vi "ADO Fields Get Count.vi"(8 "error in (no error)":errorcluster, 11 "Fields In":refnum<k7>) -> (0 "error out":errorcluster, 2 "Count":i32, 3 "Fields Out":refnum<k7>)   [LabVIEW 2013]
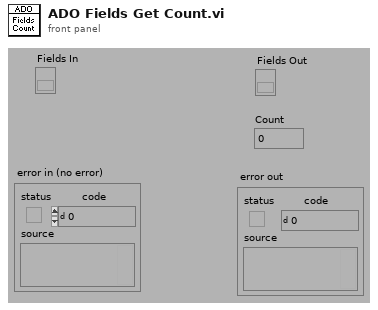
[diagram p1: front panel]
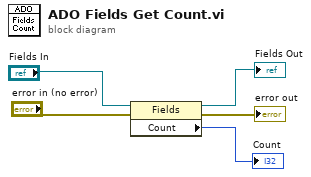
[diagram p0: block diagram]
diagram:
  n1 = property class="Fields"(reference="Fields In", error in="error in (no error)") -> (reference out=→"Fields Out":refnum<k7>, error out=→"error out":errorcluster, "Count"=→"Count":i32)
